vi "Pantalla HMI.vi"() -> ()   [LabVIEW 2021]
panel:
  in  "Limpiar Gráfica 4":bool
  in  "Limpiar Gráfica 3":bool
  in  "Limpiar Gráfica 2":bool
  out "Coordenadas (x,y)":string
  out "Image":T1(plugin-control)
  out "Mensajes":string
  in  "Puerto":refnum<visa-resource-name>
  out "date/time string":string
  out "Estable":bool
  out "Leyendo":bool
  out "Prendido":bool
  out "Suspendido":bool
  in  "Paro de emergencia":bool
  in  "Posiciones del balancín":bool
  in  "Reposo":bool
  in  "Limpiar Gráfica":bool
  in  "Encender":bool
  # "Sistema de monitoreo y control del Baymax"
  # "Comandos principales"
  # "Alarma y mensajes"
  # "Fecha y hora"
  # "Estados del proceso"
  # "Posicion actual del robot"
  # "Comandos secundarios"
  # "Configuración de comunicacion"
  # "Estadisticas"
  # "Configuración de ruta"
  # "Paro de emergencia"
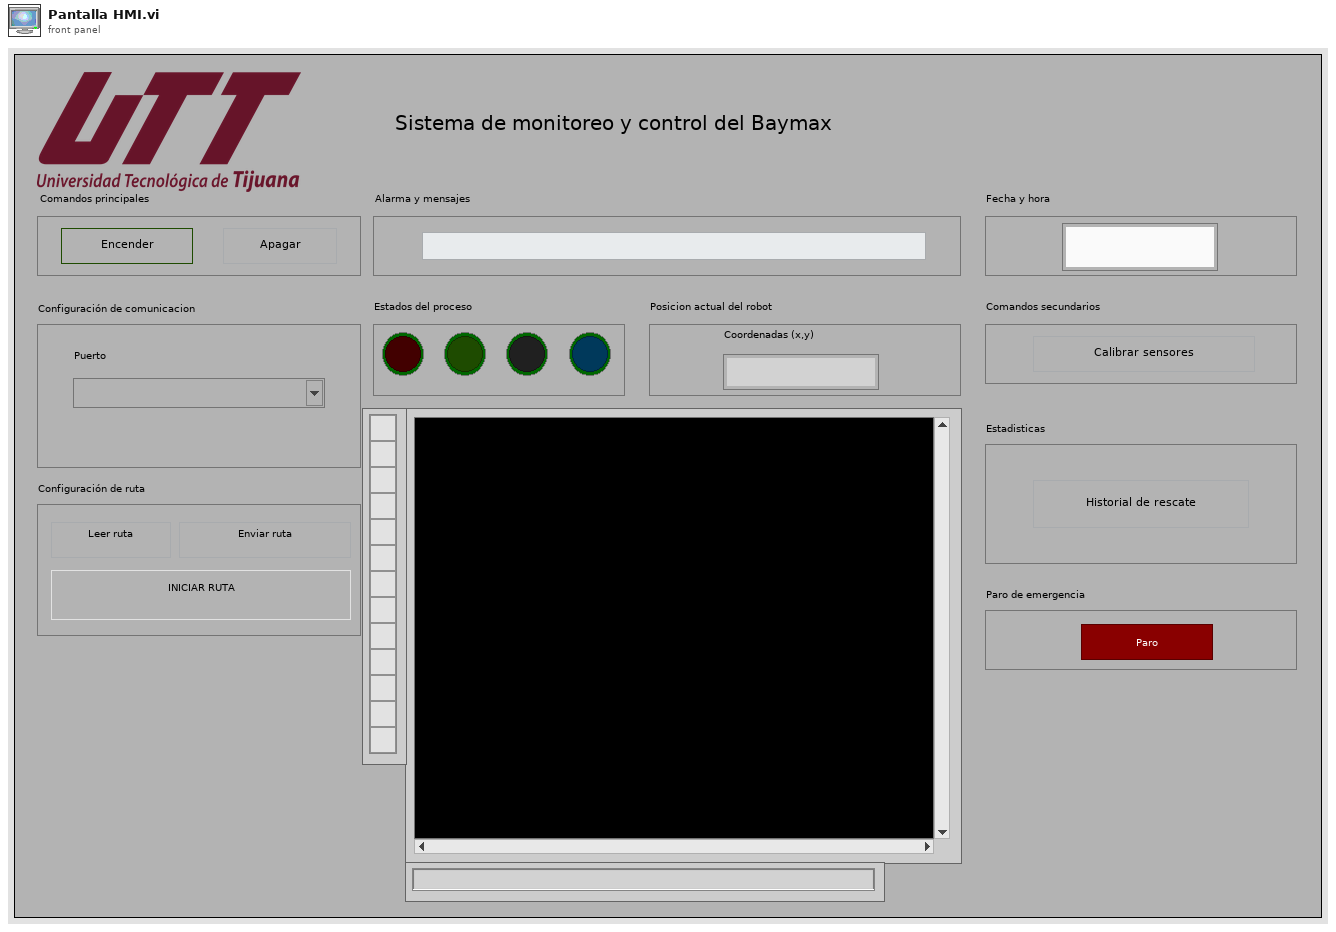
[diagram p1: front panel]
types:
  T1 = typedef "IMAQ Image.ctl" = refnum<image>
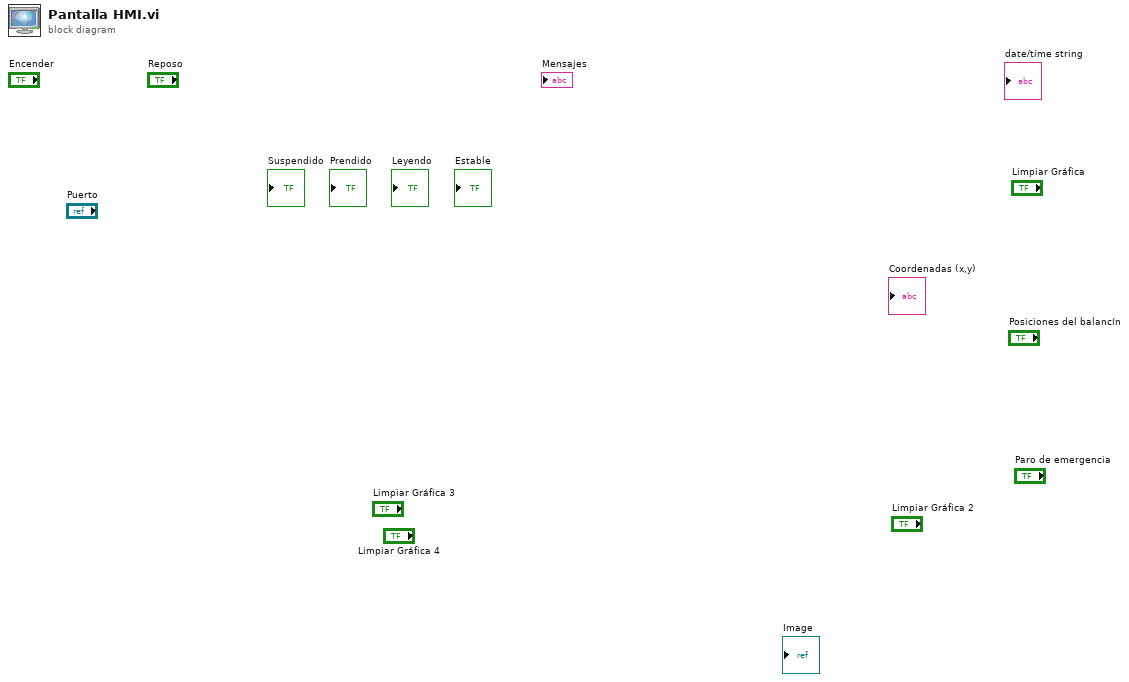
[diagram p0: block diagram]
diagram:
